vi "Ramp PSU to Target.vi"(6 "Axis":T1=enum."Z", 8 "error in (no error)":errorcluster, 9 "Target Rate (T/min)":dbl, 10 "Target Field (T)":dbl, 11 "Instrument.OxfordVRM in":refnum<class "Instrument.OxfordVRM.lvclass">) -> (0 "error out":errorcluster, 3 "Instrument.OxfordVRM out":refnum<class "Instrument.OxfordVRM.lvclass">)   [LabVIEW 2019, in "Instrument.OxfordVRM.lvclass"]
uses:
  Instrument.OxfordVRM.lvclass
  <instrlib>/Mercury iXX/Public/Libraries/Magnet/Controls/PSU Actions.ctl
  <instrlib>/Mercury iXX/Public/Libraries/Magnet.lvlib
  <userlib>/LevyLab/Instrument Framework/Instrument Types/Cryostat/Typedefs/Magnet Axis--Enum.ctl
  <userlib>/LevyLab/Instrument Framework/Instrument Types/Cryostat/Instrument.Cryostat.lvclass
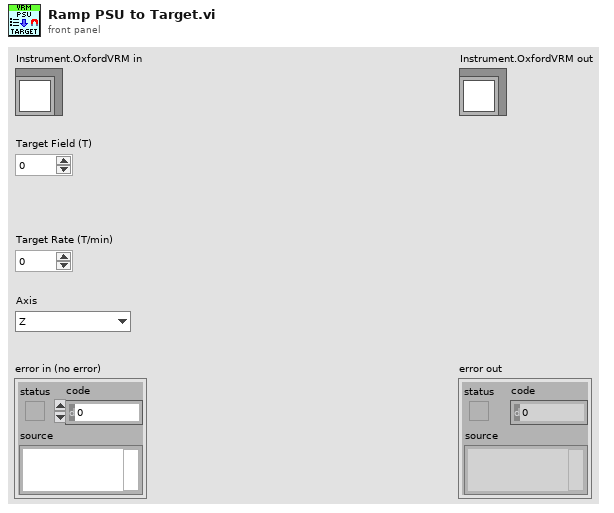
[diagram p1: front panel]
types:
  T1 = typedef "Instrument.Cryostat.lvclass/Magnet Axis--Enum.ctl" = enum16{"X", "Y", "Z"}
  T2 = typedef "Mercury iXX.lvlib/Magnet.lvlib/PSU Actions.ctl" = string
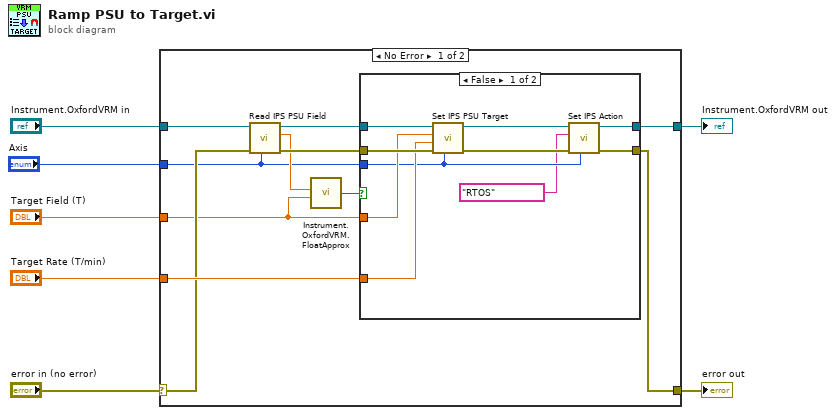
[diagram p0: block diagram]
diagram:
  n1 = case shown="No Error" "error in (no error)" {
    selector: "error in (no error)" -> [w12 w32]
    tunnel: [w15 w32] -> w6
    tunnel: [w18 w31] -> w4
    tunnel: "Instrument.OxfordVRM in" -> [w14 w31]
    tunnel: "Target Field (T)" -> [w8 _]
    tunnel: "Target Rate (T/min)" -> [w16 _]
    tunnel: "Axis" -> [w9 _]
    frame No Error {
      n2 = call "Read IPS PSU Field.vi"("Axis"=w9, "error in (no error)"=w12, "Instrument.OxfordVRM in"=w14) -> ("error out"=w11:errorcluster, "Power Supply Field (T)"=w10:dbl, "Instrument.OxfordVRM out"=w13:refnum<class "Instrument.OxfordVRM.lvclass">)  [unwired: 6 in]
      n3 = call "Instrument.OxfordVRM.FloatApprox.vi"("y"=w8, "x"=w10) -> ("x ~ y?"=w17:bool)  [unwired: 4 in]
      n4 = case shown="False" w17 {
        tunnel: [w28 w30] -> w18
        tunnel: [w27 w29] -> w15
        tunnel: w13 -> [w26 w30]
        tunnel: w11 -> [w24 w29]
        tunnel: w8 -> [w21 _]
        tunnel: w16 -> [w22 _]
        tunnel: w9 -> [w20 _]
        frame False {
          n5 = call "Set IPS PSU Target.vi"("Axis"=w20, "error in (no error)"=w24, "Target Field Rate (T/min)"=w22, "Target Field (T)"=w21, "Instrument.OxfordVRM in"=w26) -> ("error out"=w23:errorcluster, "Instrument.OxfordVRM out"=w25:refnum<class "Instrument.OxfordVRM.lvclass">)  [unwired: 4 in, 1 out]
          n6 = call "Set IPS Action.vi"("Axis"=w20, "error in (no error)"=w23, "PSU Act Stat"=T2 "RTOS", "Instrument.OxfordVRM in"=w25) -> ("error out"=w27:errorcluster, "Instrument.OxfordVRM out"=w28:refnum<class "Instrument.OxfordVRM.lvclass">)  [unwired: 5 in, 1 out]
        }
        frame True {
          # "If PSU Field == Target, do nothing"
        }
      }
    }
    frame Error {
    }
  }
  "error out" <- w6
  "Instrument.OxfordVRM out" <- w4
